vi "Left Select Beacon Loop (SubVI).vi"   [LabVIEW 2015]
uses:
  Left Variables.vi
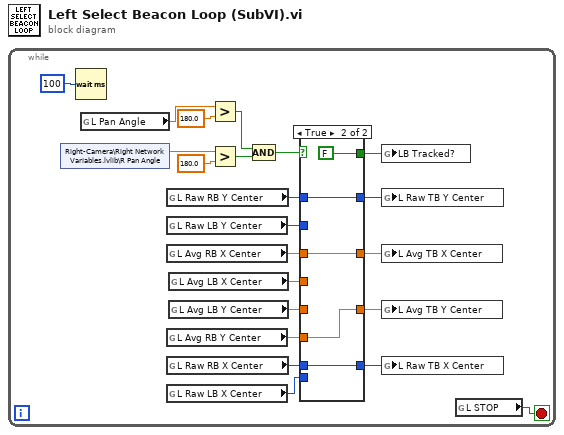
[diagram p0: block diagram]
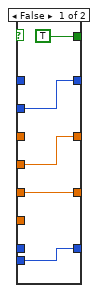
[diagram p2: hidden frame]
diagram:
  n1 = while {
    stop <- w9 stop-if-true
    n2 = shared-variable "Right-Camera\\Right Network Variables.lvlib\\R Pan Angle"() -> (w13:dbl)  [unwired: 1 in, 1 out]
    n3 = Wait (ms)(milliseconds to wait=u32 100) -> ()  [unwired: 1 out]
    n4 = global read "Left Variables.vi" "L Pan Angle"() -> (w10:dbl)
    n5 = global read "Left Variables.vi" "L Raw RB Y Center"() -> (w3:u16)
    n6 = global read "Left Variables.vi" "L Raw LB Y Center"() -> (w2:u16)
    n7 = global read "Left Variables.vi" "L Avg RB X Center"() -> (w18:dbl)
    n8 = global read "Left Variables.vi" "L Avg RB Y Center"() -> (w6:dbl)
    n9 = global read "Left Variables.vi" "L Raw RB X Center"() -> (w20:u16)
    n10 = global read "Left Variables.vi" "L Raw LB X Center"() -> (w19:u16)
    n11 = global read "Left Variables.vi" "L Avg LB X Center"() -> (w17:dbl)
    n12 = global read "Left Variables.vi" "L Avg LB Y Center"() -> (w7:dbl)
    n13 = Greater?(x=w10, y=180.0 ("upper limit")) -> (0:w15:bool)
    n14 = Greater?(x=w13, y=180.0 ("upper limit")) -> (0:w14:bool)
    n15 = Compound Arithmetic op=AND(w15, w14) -> (w16:bool)
    n16 = case shown="True" w16 {
      tunnel: [w27 w32] -> w22
      tunnel: w20 -> [_ w32]
      tunnel: w19 -> [w27 _]
      tunnel: [w26 w31] -> w21
      tunnel: w17 -> [w26 _]
      tunnel: w18 -> [_ w31]
      tunnel: [w25 w30] -> w5
      tunnel: w7 -> [w25 _]
      tunnel: w6 -> [_ w30]
      tunnel: [w24 w29] -> w4
      tunnel: w3 -> [_ w29]
      tunnel: w2 -> [w24 _]
      tunnel: [TRUE FALSE] -> w1
      frame False {
      }
      frame True {
      }
    }
    n17 = global write "Left Variables.vi" "LB Tracked?"(w1) -> ()
    n18 = global write "Left Variables.vi" "L Raw TB Y Center"(w4) -> ()
    n19 = global write "Left Variables.vi" "L Avg TB X Center"(w21) -> ()
    n20 = global write "Left Variables.vi" "L Avg TB Y Center"(w5) -> ()
    n21 = global write "Left Variables.vi" "L Raw TB X Center"(w22) -> ()
    n22 = global read "Left Variables.vi" "L STOP"() -> (w9:bool)
  }
